vi "Random Number Nested.vi"(11 "Hello World Event in":refnum<class "Hello World Event.lvclass">) -> ()   [LabVIEW 2021, in "Hello World Event.lvlib" / "Hello World Event.lvclass"]
uses:
  Hello World Event.lvclass
  Hello World Event.lvclass/Hello World Event.ctl
  <vilib>/numeric/Random Number (Range) U64.vi
  <vilib>/numeric/sub_Random U32.vi
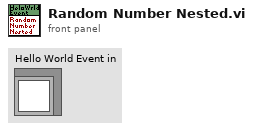
[diagram p1: front panel]
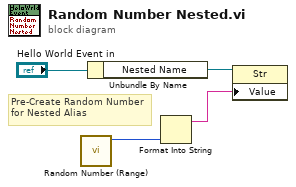
[diagram p0: block diagram]
diagram:
  # "Pre-Create Random Number for Nested Alias"
  n1 = call-poly <vilib>:"Random Number (Range).vi"() -> ("number"=w4:u64)  [unwired: 11 in]
  n2 = Unbundle By Name("Hello World Event in") -> ("Nested Name"=w1:refnum<vi>)
  n3 = Format Into String(w4) -> (resulting string=w3:string)  [unwired: 3 in, 1 out]
  n4 = property class="Str"(reference=w1, "Value"=w3) -> ()  [unwired: 1 in, 2 out]
